vi "Insight String Package.vi"(2 "Footer":string, 3 "String":string, 4 "Header":string) -> (0 "resulting string":string)   [LabVIEW 2013]
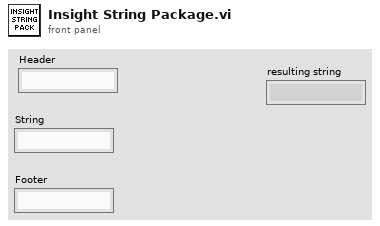
[diagram p1: front panel]
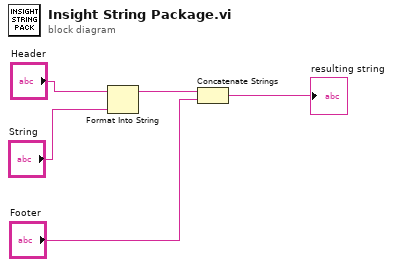
[diagram p0: block diagram]
diagram:
  n1 = Format Into String(initial string="Header", "String") -> (resulting string=w2:string)  [unwired: 2 in, 1 out]
  n2 = Concatenate Strings(w2, "Footer") -> (→"resulting string":string)
